vi "Format IamInstanceProfileResponseType_LVXML.vi"(8 "error in (no error)":errorcluster, 11 "xmlData in":T2) -> (0 "error out":errorcluster, 3 "IamInstanceProfileResponseType":T3)   [LabVIEW 2014, in "AWS_EC2.lvlib" / "AWS_EC2.lvclass"]
uses:
  AWS_EC2.lvclass
  EC2 Datatypes/IamInstanceProfileResponseType.ctl
  lv-xml-parser/r0/trunk/VI Source/EventType.ctl
  AWS_EC2.lvlib
  lv-xml-parser/r0/trunk/VI Source/LV XML Parser.lvlib
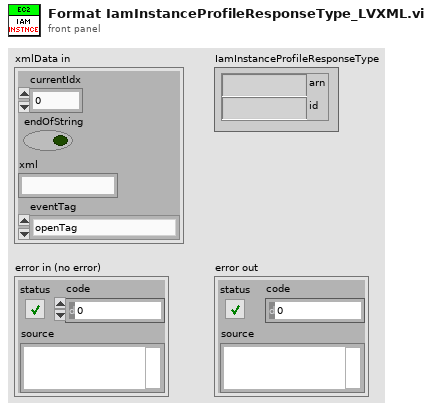
[diagram p1: front panel]
types:
  T1 = typedef "LV XML Parser.lvlib/EventType.ctl" = enum16{"openTag", "endOpenTag", "closeTag", "comment", "endComment", "endOfFile", "attribute", "startXml"}
  T2 = cluster{"currentIdx":i32, "endOfString":bool, "xml":string, "eventTag":T1}
  T3 = typedef "AWS_EC2.lvlib/IamInstanceProfileResponseType.ctl" = cluster{"arn":string, "id":string}
  T4 = cluster{"namespaceUri":string, "localName":string}
  T5 = cluster{"Attributes":cluster{"localName":string, "namespaceUri":string, "value":string}[], "localName":string, "namespaceUri":string, "valueXmlData":cluster{"currentIdx":i32, "endOfString":bool, "xml":string, "eventTag":T1}}[]
  T6 = cluster{"Attributes":cluster{"localName":string, "namespaceUri":string, "value":string}[], "localName":string, "namespaceUri":string, "valueXmlData":cluster{"currentIdx":i32, "endOfString":bool, "xml":string, "eventTag":T1}}
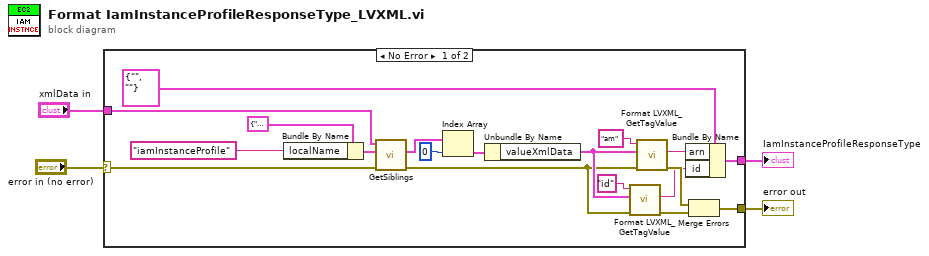
[diagram p0: block diagram]
diagram:
  n1 = case shown="No Error" "error in (no error)" {
    selector: "error in (no error)" -> [w15 w24]
    tunnel: "xmlData in" -> [w16 _]
    tunnel: [w6 w24] -> w2
    tunnel: [w13 _] -> w4
    frame No Error {
      n2 = Bundle By Name(cluster=T4 {"namespaceUri"="", "localName"=""} ("limitToTag"), "localName"="iamInstanceProfile" ("Tag name")) -> (w22:T4)
      n3 = call "GetSiblings.vi"("error in (no error)"=w15, "limitToTag"=w22, "xmlData"=w16) -> ("error out"=w9:errorcluster, "Siblings"=w19:T5)  [unwired: 7 in]
      n4 = Index Array(array=w19, index=0) -> (element=w18:T6)
      n5 = Unbundle By Name(w18) -> ("valueXmlData"=w10:T2)
      n6 = call "Format LVXML_GetTagValue.vi"("error in (no error)"=w9, "xmlDataIn"=w10, "Tag name"="id") -> ("error out"=w8:errorcluster, "Value"=w5:string)  [unwired: 6 in, 1 out]
      n7 = call "Format LVXML_GetTagValue.vi"("error in (no error)"=w9, "xmlDataIn"=w10, "Tag name"="am") -> ("error out"=w7:errorcluster, "Value"=w12:string)  [unwired: 6 in, 1 out]
      n8 = Bundle By Name(cluster=T3 {"arn"="", "id"=""} ("IamInstanceProfileResponseType"), "arn"=w12, "id"=w5) -> (w13:T3)
      n9 = Merge Errors(w7, w8) -> (w6:errorcluster)
    }
    frame Error {
    }
  }
  "IamInstanceProfileResponseType" <- w4
  "error out" <- w2
